vi "CPP_CalcTubingCorrection.vi"() -> (5 "Plug in titles":string[](array[string]), 7 "Plug in values":string[](array[string]))   [LabVIEW 2016]
uses:
  <vilib>/Analysis/baseanly.llb/Mean (DBL).vi
  Globals/Meas_global.vi
  <vilib>/Analysis/NI_AALBase.lvlib
  <vilib>/Analysis/NI_AALPro.lvlib
panel:
  in  "Tab Control":enum32{"TubingCorrection", "Setup"}(tab)
  in  "RefXducer":i32(ring) items=["Mano (Pref)", "Mano (1)", "Mano (2)", "Mano (3)", "Mano (4)", "Mano (5)", "Mano (6)", "Mano (7)", "Mano (8)", "Mano (9)", "Mano (10)", "Mano (11)", "Mano (12)", "Mano (PitotLocal)", "RV (5V)", "RV (Ch23)"]
  in  "TestXducer":i32(ring) items=["Mano (Pref)", "Mano (1)", "Mano (2)", "Mano (3)", "Mano (4)", "Mano (5)", "Mano (6)", "Mano (7)", "Mano (8)", "Mano (9)", "Mano (10)", "Mano (11)", "Mano (12)", "Mano (PitotLocal)", "RV (5V)", "RV (Ch23)"]
  out "Time Traces":cluster{dbl, dbl, dbl[][]}(graph)
  out "Spectra":cluster{dbl, "df (Hz)":dbl, dbl[][]}(graph)
  in  "stop":bool
  in  "Pause Button":bool
  in  "Pause(ms)":u32=500
  in  "Coherence Threshold":dbl=0.98
  out "Coefficients Smoothed and Normalized":bool
  in  "Decimate Correction File?":bool=TRUE
  in  "Smooth Correction File?":bool=TRUE
  in  "CorrectionFileDestinationPath":path
  in  "fcut (Hz)":dbl=1000.0
  in  "Cutoff type":string(combo)="Brickwall"
  out "SD(boosted)":dbl format="%.3e"
  out "SD(ref)":dbl format="%.3e"
  out "SD(Boostederror%)":dbl format="%#_3g"
  out "Current Block No":i32
  in  "LowFrequencySmoothingFloor":dbl=3.0
  in  "LowFrequencySmoothingCeiling":dbl=7.0
  in  "ExistingTubingCorrectionFile":path
  in  "Apply Phase Correction?":bool=TRUE
  in  "Save Files?":bool
  in  "Use Existing Correction File?":bool
  out "df (Hz)":dbl format="%.6f"
  in  "Decimation Term":i32=10
  out "OutputString":string
  in  "N Points To Average Either Side":i32=10
  in  "Force Phase 0 Intercept?":bool=TRUE
  out "SD(muted)":dbl format="%.3e"
  out "SD(Mutederror%)":dbl format="%#_3g"
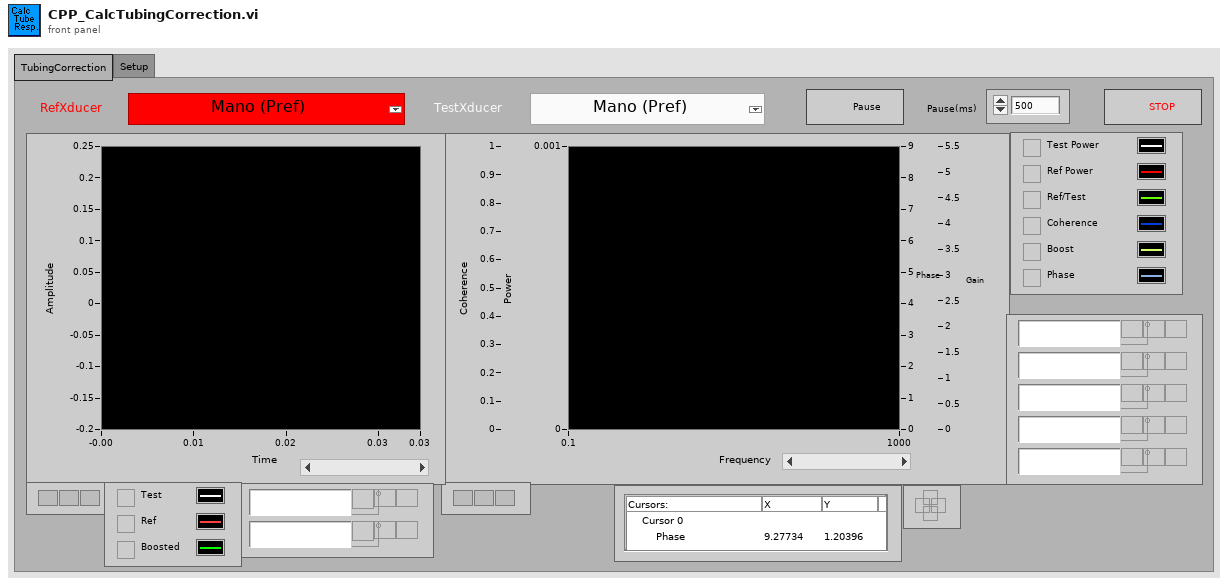
[diagram p1: front panel]
types:
  T1 = typedef "Analysis_info_cluster.ctl" = cluster{"Colour":u32, "Inst type":T2, "Inst name":string, "Symbol":string, "Code name":string, "Extra Info":string, "Inst Array":T3, "Extra Titles":string[], "Extra Values":string[], "U":dbl, "u^2":dbl, "u^3":dbl, "u^4":dbl, "Skew_u":dbl, "Kurt_u":dbl, "Sd Error in Mean":dbl, "% u'/U":dbl, "X":dbl, "Y":dbl, "Z":dbl, "Timescale integral to 25%":dbl, "Sd Error in Variance":dbl, "Calib File":path, "Calib Constants":dbl[], "Output Position":bool, "Full Stats":bool, "Av Sampling Rate":dbl, "Av No of Samples":dbl, "Total Meas Time (s)":dbl, "ADAM Ch Name":string, "Max value":dbl, "Min value":dbl}
  T2 = typedef "Inst_type.ctl" = enum16{"Propeller anemometer", "Raw voltage", "Pressure Transducer", "Pitot-static tube", "Preston tube", "Hot wire", "Cross wire 1", "Cross wire 2", "Generic Linear", "Generic Polynomial", "Generic BackPoly", "Fast FID", "Thermocouple", "Cold wire", "Pulsed Wire", "LDA Vel", "LDA Tran time", "LDA Arr time", "Microphone"}
  T3 = typedef "Instrument_Array.ctl" = enum16{"PWA", "LDA", "Analogue"}
  T4 = typedef "Time_Trace_Cluster.ctl" = cluster{"Weighting":dbl[], "Time (s)":dbl[], "Voltage":dbl[], "Eng Values":dbl[]}
  T5 = enum16{"open", "replace", "create", "open or create", "replace or create", "replace or create with confirmation"}
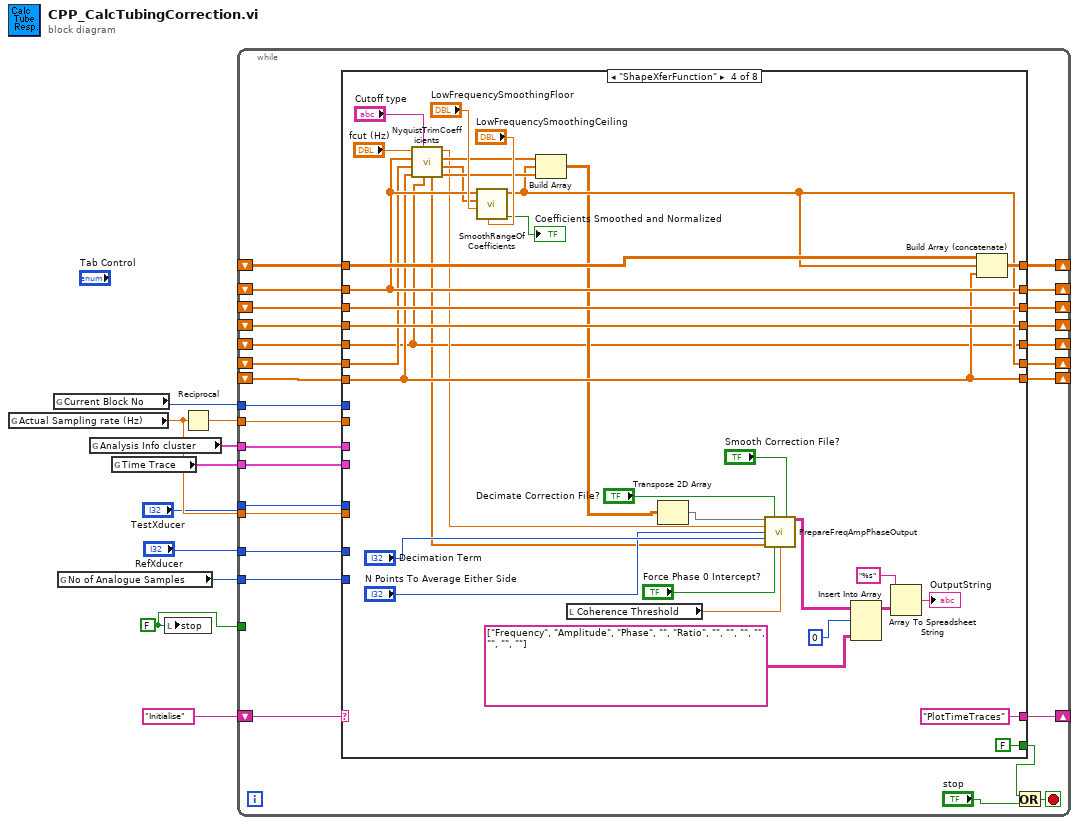
[diagram p0: block diagram]
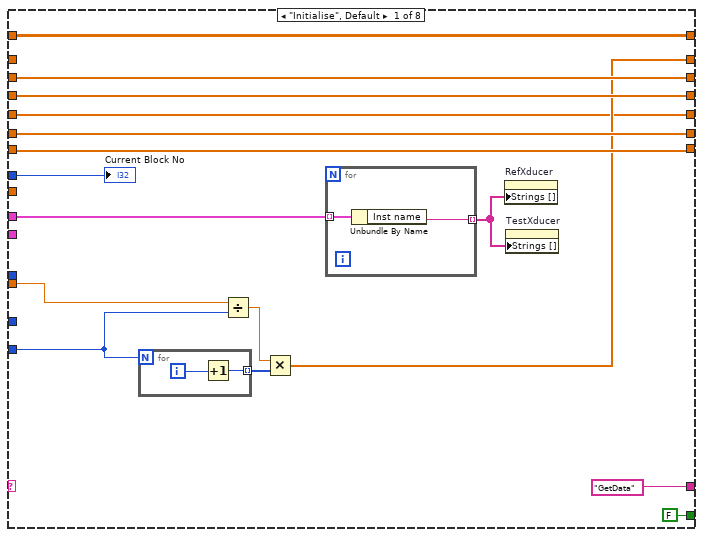
[diagram p2: hidden frame]
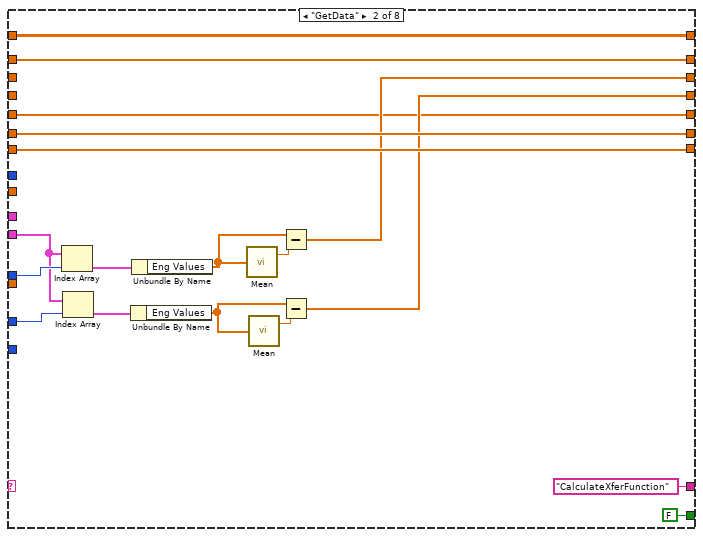
[diagram p3: hidden frame]
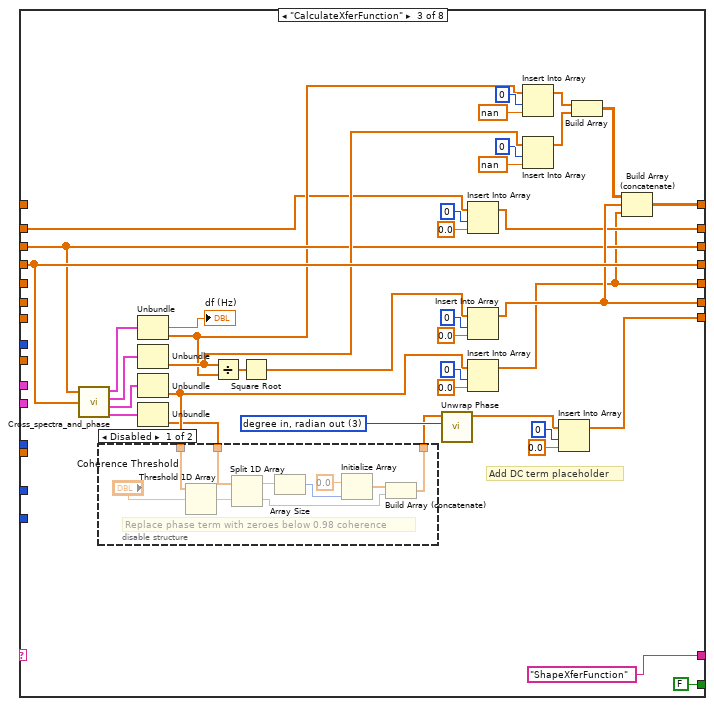
[diagram p4: hidden frame]
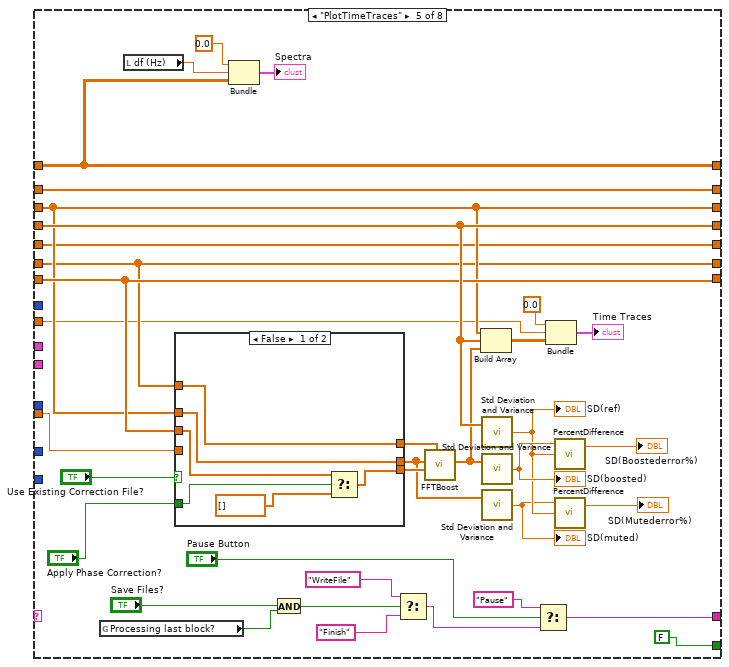
[diagram p6: hidden frame]
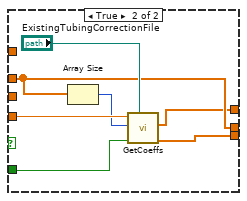
[diagram p7: hidden frame]
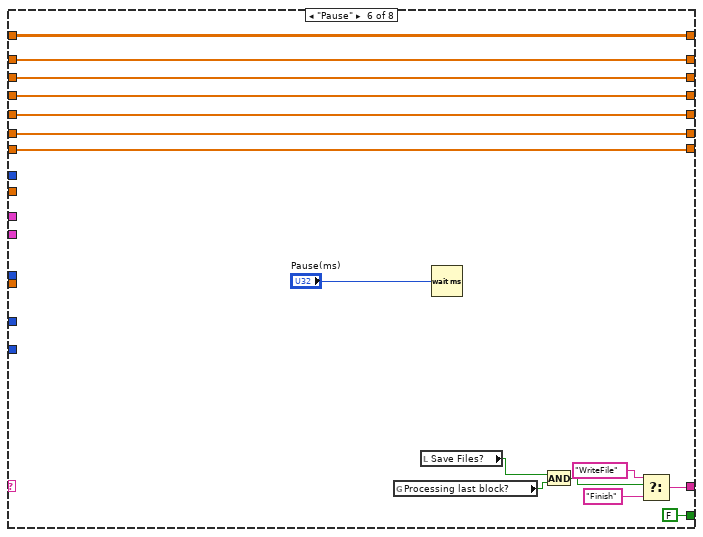
[diagram p8: hidden frame]
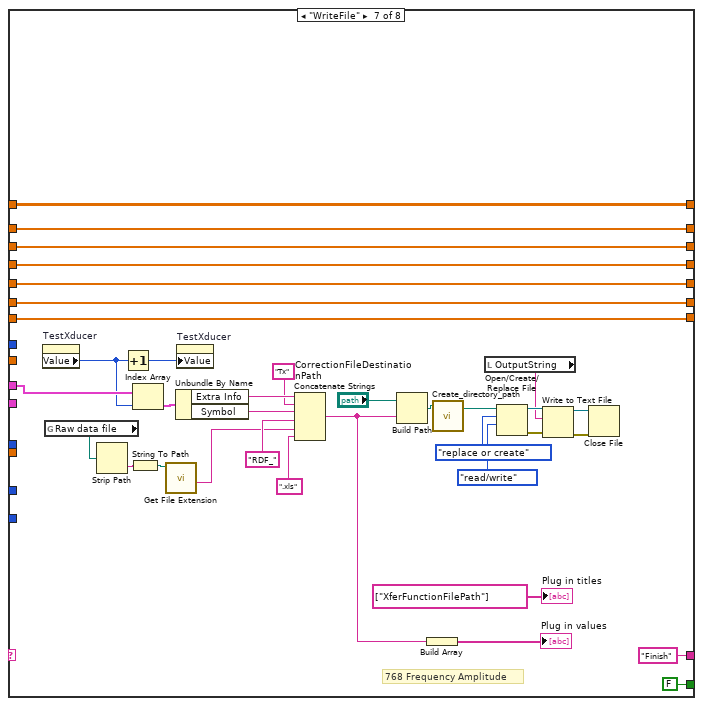
[diagram p9: hidden frame]
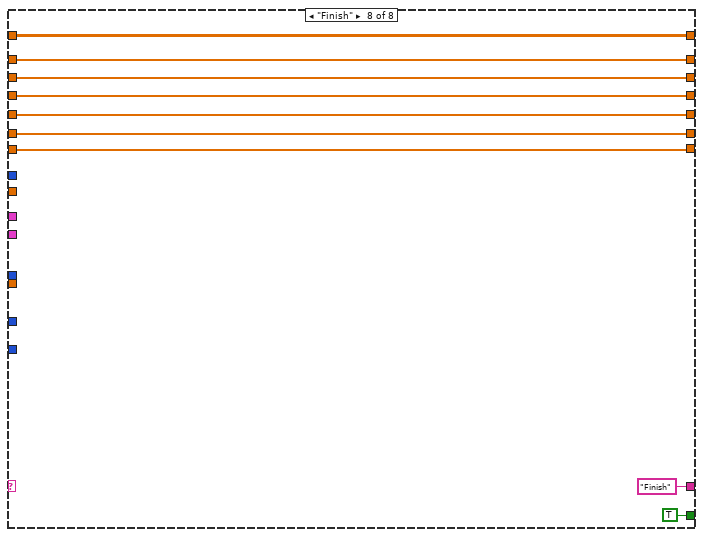
[diagram p10: hidden frame]
diagram:
  w9 = FALSE ("stop")
  n1 = global read "Meas_global.vi" "Actual Sampling rate (Hz)"() -> (w3:dbl)
  n2 = global read "Meas_global.vi" "Current Block No"() -> (w7:i32)
  n3 = global read "Meas_global.vi" "No of Analogue Samples"() -> (w2:i32)
  n4 = global read "Meas_global.vi" "Analysis Info cluster"() -> (w6:T1[])
  n5 = global read "Meas_global.vi" "Time Trace"() -> (w5:T4[])
  n6 = local write "stop"(w9) -> ()
  n7 = Reciprocal(x=w3) -> (1/x=w4:dbl)
  n8 = while {
    shift-right: [w33] -> _
    shift-left: "Initialise" -> [w37]
    tunnel: w6 -> [w36]
    tunnel: "RefXducer" -> [w34]
    tunnel: w4 -> [w32]
    tunnel: w9 -> [_]
    shift-right: [w31] -> _
    shift-left: _ -> [w29]
    shift-right: [w30] -> _
    shift-left: _ -> [w28]
    tunnel: w7 -> [w27]
    tunnel: w5 -> [w26]
    shift-right: [w25] -> _
    shift-left: _ -> [w24]
    tunnel: w3 -> [w23]
    shift-right: [w22] -> _
    shift-left: _ -> [w21]
    tunnel: w2 -> [w20]
    shift-right: [w19] -> _
    shift-left: _ -> [w18]
    shift-right: [w17] -> _
    shift-left: _ -> [w16]
    tunnel: "TestXducer" -> [w35]
    shift-right: [w12] -> _
    shift-left: _ -> [w11]
    stop <- w14 stop-if-true
    n9 = case shown="\"ShapeXferFunction\"" w37 {
      tunnel: w36 -> [w49 _ _ _ _ _ w239 _]
      tunnel: w35 -> [_ w75 _ _ _ _ _ _]
      tunnel: w34 -> [_ w74 _ _ _ _ _ _]
      tunnel: ["GetData" "CalculateXferFunction" "ShapeXferFunction" ("t") "PlotTimeTraces" ("t") w193 w214 "Finish" ("t") "Finish" ("t")] -> w33
      tunnel: w32 -> [_ _ _ _ w168 _ _ _]
      tunnel: [w52 w61 w86 w160 w184 w224 w259 w268] -> w31
      tunnel: [w51 w60 w107 w159 w186 w223 w258 w267] -> w30
      tunnel: w29 -> [w52 _ w86 w160 w184 w224 w259 w268]
      tunnel: w28 -> [w51 _ w107 w159 w186 w223 w258 w267]
      tunnel: w27 -> [w50 _ _ _ _ _ _ _]
      tunnel: w26 -> [_ w70 _ _ _ _ _ _]
      tunnel: [w47 w68 w93 w137 w182 w220 w255 w264] -> w22
      tunnel: [w48 w69 w88 w149 w185 w221 w256 w265] -> w25
      tunnel: w24 -> [w48 w69 _ w149 w185 w221 w256 w265]
      tunnel: w23 -> [w46 _ _ _ w167 _ _ _]
      tunnel: w21 -> [w47 w68 _ w150 w182 w220 w255 w264]
      tunnel: w20 -> [w45 _ _ _ _ _ _ _]
      tunnel: [w44 w67 w81 w151 w183 w219 w254 w263] -> w19
      tunnel: w18 -> [_ w67 w82 w151 w183 w219 w254 w263]
      tunnel: [w43 w66 w114 w155 w189 w218 w253 w262] -> w17
      tunnel: w16 -> [w43 w66 _ w156 w189 w218 w253 w262]
      tunnel: [FALSE FALSE FALSE FALSE FALSE FALSE FALSE TRUE] -> w13
      tunnel: [w38 w58 w76 w128 w165 w210 w230 w260] -> w12
      tunnel: w11 -> [w38 w58 _ w128 w165 w210 w230 w260]
      frame "Initialise", Default {
        n10 = for {
          N: w45 -> [_]
          tunnel: [w54] -> w41 mode=indexing
          i -> [w55]
          n11 = Increment(x=w55) -> (x+1=w54:i32)
        }
        n12 = Divide(x=w46, y=w45) -> (x/y=w40:dbl)
        n13 = Multiply(x=w40, y=w41) -> (x*y=w44:dbl[])
        n14 = for {
          tunnel: w49 -> [w57] mode=indexing
          tunnel: [w56] -> w42 mode=indexing
          n15 = Unbundle By Name(w57) -> ("Inst name"=w56:string)
        }
        n16 = property on="RefXducer" class="Ring (strict)"("Strings []"=w42) -> ()  [unwired: 2 in, 2 out]
        n17 = property on="TestXducer" class="Ring (strict)"("Strings []"=w42) -> ()  [unwired: 2 in, 2 out]
        "Current Block No" <- w50
      }
      frame "GetData" {
        n18 = Index Array(array=w70, index=w75) -> (element=w72:T4)
        n19 = Index Array(array=w70, index=w74) -> (element=w71:T4)
        n20 = Unbundle By Name(w71) -> ("Eng Values"=w62:dbl[])
        n21 = Unbundle By Name(w72) -> ("Eng Values"=w63:dbl[])
        n22 = call-poly <vilib>:"Mean.vi"("X"=w63) -> ("mean"=w64:dbl)  [unwired: 1 out]
        n23 = call-poly <vilib>:"Mean.vi"("X"=w62) -> ("mean"=w65:dbl)  [unwired: 1 out]
        n24 = Subtract(x=w63, y=w64) -> (x-y=w61:dbl[])
        n25 = Subtract(x=w62, y=w65) -> (x-y=w60:dbl[])
      }
      frame "CalculateXferFunction" {
        w109 = 3 items=["radian in, radian out", "radian in, degree out", "degree in, degree out", "degree in, radian out"] ("phase unit")
        # "Add DC term placeholder"
        n26 = call "Cross_spectra_and_phase.vi"("U1"=w86, "U2"=w107) -> ("U1 spectra"=w113:cluster{dbl, dbl, dbl[]}, "U2 spectra"=w112:cluster{dbl, dbl, dbl[]}, "U1 U2 coherence"=w111:cluster{dbl, dbl, "Coherence array":dbl[]}, "U1 U2 phase"=w110:cluster{dbl, dbl, "Phase array":dbl[]})  [unwired: 3 out]
        n27 = Unbundle(w113) -> (→"df (Hz)":dbl, w85:dbl[])  [unwired: 1 out]
        n28 = Unbundle(w112) -> (w97:dbl[])  [unwired: 2 out]
        n29 = Unbundle(w111) -> ("Coherence array"=w80:dbl[])  [unwired: 2 out]
        n30 = Unbundle(w110) -> ("Phase array"=w79:dbl[])  [unwired: 2 out]
        n31 = disable-structure shown="Disabled" {
          disable-tunnel: w80 -> [w124 _]
          disable-tunnel: w79 -> [w122 w125]
          disable-tunnel: [w117 w125] -> w78
          frame Disabled {
            # "Replace phase term with zeroes below 0.98 coherence"
            n32 = Threshold 1D Array(2:"Coherence Threshold", 3:w124) -> (0:w123:dbl)  [unwired: 1 in]
            n33 = Split 1D Array(array=w122, index=w123) -> (first subarray=w121:dbl[], second subarray=w120:dbl[])
            n34 = Array Size(array=w121) -> (size(s)=w119:i32)
            n35 = Initialize Array(0.0 ("element"), w119) -> (w118:dbl[])
            n36 = Build Array (concatenate)(w118, w120) -> (w117:dbl[])
          }
          frame Enabled {
          }
        }
        n37 = Divide(x=w97, y=w85) -> (x/y=w105:dbl[])
        n38 = Square Root(x=w105) -> (sqrt(x)=w94:dbl[])
        n39 = call <vilib>:"Unwrap Phase.vi"("phase unit"=w109, "Phase"=w78) -> ("Unwrapped Phase"=w77:dbl[])  [unwired: 8 in, 1 out]
        n40 = Insert Into Array(array=w82, index=0, new element=0.0 ("new element/subarray")) -> (w81:dbl[])
        n41 = Insert Into Array(array=w94, index=0, new element=0.0 ("new element/subarray")) -> (w93:dbl[])
        n42 = Insert Into Array(array=w80, index=0, new element=0.0 ("new element/subarray")) -> (w76:dbl[])
        n43 = Insert Into Array(array=w85, index=0, new element=nan ("new element/subarray")) -> (w99:dbl[])
        n44 = Insert Into Array(array=w97, index=0, new element=nan ("new element/subarray")) -> (w98:dbl[])
        n45 = Insert Into Array(array=w77, index=0, new element=0.0 ("new element/subarray")) -> (w88:dbl[])
        n46 = Build Array(w99, w98) -> (w106:dbl[][])
        n47 = Build Array (concatenate)(w106, w93, w76) -> (w114:dbl[][])
      }
      frame "ShapeXferFunction" {
        n48 = call "NyquistTrimCoefficients.vi"("Coherence"=w128, "Cutoff type"="Cutoff type", "InterpolatedPhase"=w149, "InterpolatedCoefficients"=w150, "Frequencies"=w151, "fcut (Hz)"="fcut (Hz)") -> ("NyquistLimitedPhase"=w141:dbl[], "NyquistLimitedCoefficients"=w140:dbl[], "NyquistLimitedFrequency"=w139:dbl[], "fcut Index"=w136:dbl, "NyquistLimitedCoherence"=w127:dbl[])  [unwired: 1 in]
        n49 = call "SmoothRangeOfCoefficients.vi"("LFSmoothingCeiling"="LowFrequencySmoothingCeiling", "LFSmoothingFloor"="LowFrequencySmoothingFloor", "NyquistLimitedCoefficients In"=w140, "Frequencies In"=w151) -> ("Coefficients Smoothed and Normalized"=→"Coefficients Smoothed and Normalized":bool, "NyquistLimitedCoefficients Out"=w137:dbl[])  [unwired: 5 in, 1 out]
        n50 = Build Array(w139, w137, w141) -> (w133:dbl[][])
        n51 = local read "Coherence Threshold"() -> (w126:dbl)
        n52 = Transpose 2D Array(2D array=w133) -> (transposed array=w132:dbl[][])
        n53 = call "PrepareFreqAmpPhaseOutput.vi"("Array in"=w132, "Decimate Correction File?"="Decimate Correction File?", "Smooth Correction File?"="Smooth Correction File?", "fcut Index"=w136, "N Points To Average Either Side"="N Points To Average Either Side", "Decimation Term"="Decimation Term", "Coherence"=w127, "Force Phase 0 Intercept?"="Force Phase 0 Intercept?", "Coherence Threshold"=w126) -> ("Array out"=w143:string[][])  [unwired: 6 in]
        n54 = Insert Into Array(array=w143, index (row)=0, new element=string[][] [["Frequency", "Amplitude", "Phase"], ["", "Ratio", ""], ["", "", ""], ["", "", ""]]) -> (w145:string[][])  [unwired: 1 in]
        n55 = Array To Spreadsheet String(array=w145, 3:"%s" ("format string")) -> (spreadsheet string=→"OutputString":string)  [unwired: 1 in]
        n56 = Build Array (concatenate)(w156, w137, w149) -> (w155:dbl[][])
      }
      frame "PlotTimeTraces" {
        n57 = global read "Meas_global.vi" "Processing last block?"() -> (w176:bool)
        n58 = local read "df (Hz)"() -> (w172:dbl)
        n59 = case shown="False" "Use Existing Correction File?" {
          tunnel: w185 -> [w199 _]
          tunnel: w184 -> [w202 w206]
          tunnel: w182 -> [w201 _]
          tunnel: w167 -> [_ w208]
          tunnel: [w201 w205] -> w171
          tunnel: [w202 w206] -> w164
          tunnel: [w197 w204] -> w170
          tunnel: "Apply Phase Correction?" -> [w200 w203]
          frame False {
            n60 = Select(t=w199, s=w200, f=dbl[] [] ("NyquistLimitedPhase")) -> (s? t:f=w197:dbl[])
          }
          frame True {
            n61 = Array Size(array=w206) -> (size(s)=w207:i32)
            n62 = call "GetCoeffs.vi"("PathToFile"="ExistingTubingCorrectionFile", "Apply Phase Correction?"=w203, "SignalLength"=w207, "fs (Hz)"=w208) -> ("NyquistLimitedPhase"=w204:dbl[], "NyquistLimitedCoefficients"=w205:dbl[])  [unwired: 6 in]
          }
        }
        n63 = Bundle(0.0, "df (Hz)"=w172, w189) -> (→"Spectra":cluster{dbl, "df (Hz)":dbl, dbl[][]})  [unwired: 1 in]
        n64 = And(x="Save Files?", y=w176) -> (x .and. y?=w175:bool)
        n65 = Select(t="WriteFile", s=w175, f="Finish") -> (s? t:f=w179:string)
        n66 = call "FFTBoost.vi"("CompensationCoefficients"=w171, "PhaseCorrection"=w170, "mutedData"=w164) -> ("boostedData"=w169:dbl[])  [unwired: 1 in, 7 out]
        n67 = Build Array(w184, w186, w169) -> (w192:dbl[][])
        n68 = call <vilib>:"Std Deviation and Variance.vi"("X"=w186) -> ("standard deviation"=w163:dbl)  [unwired: 1 in, 2 out]
        "SD(ref)" <- w163
        n69 = call <vilib>:"Std Deviation and Variance.vi"("X"=w169) -> ("standard deviation"=w187:dbl)  [unwired: 1 in, 2 out]
        "SD(boosted)" <- w187
        n70 = call <vilib>:"Std Deviation and Variance.vi"("X"=w164) -> ("standard deviation"=w162:dbl)  [unwired: 1 in, 2 out]
        "SD(muted)" <- w162
        n71 = Select(t="Pause", s="Pause Button", f=w179) -> (s? t:f=w193:string)
        n72 = Bundle(0.0, w168, w192) -> (→"Time Traces":cluster{dbl, dbl, dbl[][]})  [unwired: 1 in]
        n73 = call "PercentDifference.vi"("Basis"=w163, "Comparee"=w187) -> ("PercentageDifference"=→"SD(Boostederror%)":dbl)  [unwired: 1 in, 1 out]
        n74 = call "PercentDifference.vi"("Basis"=w163, "Comparee"=w162) -> ("PercentageDifference"=→"SD(Mutederror%)":dbl)  [unwired: 1 in, 1 out]
      }
      frame "Pause" {
        n75 = global read "Meas_global.vi" "Processing last block?"() -> (w212:bool)
        n76 = local read "Save Files?"() -> (w213:bool)
        n77 = Wait (ms)(milliseconds to wait="Pause(ms)") -> ()  [unwired: 1 out]
        n78 = And(x=w213, y=w212) -> (x .and. y?=w211:bool)
        n79 = Select(t="WriteFile", s=w211, f="Finish") -> (s? t:f=w214:string)
      }
      frame "WriteFile" {
        # "768 Frequency Amplitude"
        n80 = property on="TestXducer" class="Ring (strict)"() -> ("Value"=w232:i32)  [unwired: 2 in, 2 out]
        n81 = global read "Meas_global.vi" "Raw data file"() -> (w236:path)
        n82 = Strip Path(path=w236) -> (name=w235:string)  [unwired: 1 out]
        n83 = Increment(x=w232) -> (x+1=w233:i32)
        n84 = String To Path(string=w235) -> (path=w234:path)
        n85 = Index Array(array=w239, index=w232) -> (element=w238:T1)
        n86 = call <vilib>:"Get File Extension.vi"("file"=w234) -> ("filename without extension"=w225:string)  [unwired: 6 in, 4 out]
        n87 = Unbundle By Name(w238) -> ("Extra Info"=w229:string, "Symbol"=w227:string)
        n88 = property on="TestXducer" class="Ring (strict)"("Value"=w233) -> ()  [unwired: 2 in, 2 out]
        n89 = Concatenate Strings(w229, "Tx" ("string"), w227, "RDF_" ("string"), w225, ".xls" ("string")) -> (w249:string)
        n90 = Build Path(base path="CorrectionFileDestinationPath", name or relative path=w249) -> (appended path=w241:path)
        n91 = Build Array(w249) -> (→"Plug in values":string[])
        n92 = call "Create_directory_path.vi"("Path name"=w241) -> ("Path name Out"=w240:path)  [unwired: 2 in, 1 out]
        n93 = local read "OutputString"() -> (w244:string)
        n94 = Open/Create/Replace File(file path (use dialog)=w240, operation (0:open)=T5."replace or create", access (0:read/write)=enum16{"read/write", "read-only", "write-only"}."read/write") -> (refnum out=w245:refnum<file>, error out=w246:errorcluster)  [unwired: 3 in, 1 out]
        n95 = Write to Text File(file (use dialog)=w245, text=w244, error in=w246) -> (refnum out=w242:refnum<file>, error out=w243:errorcluster)  [unwired: 1 in, 1 out]
        n96 = Close File(refnum=w242, error in=w243) -> ()  [unwired: 2 out]
        "Plug in titles" <- string[] ["XferFunctionFilePath"] ("Add in values")
      }
      frame "Finish" {
      }
    }
    n97 = Or(x=w13, y="stop") -> (x .or. y?=w14:bool)
  }
